vi "Becker-Hickl Read Single SGL.vi"(8 "Error In":errorcluster, 10 "Default":sgl, 11 "Bytes in":string) -> (0 "Error Out":errorcluster, 2 "SGL":sgl, 3 "Bytes out":string)   [LabVIEW 2021, in "Becker-Hickl Files.lvlib"]
uses:
  Becker-Hickl Files.lvlib
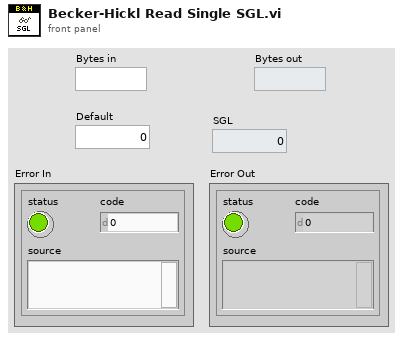
[diagram p1: front panel]
types:
  T1 = enum16{"big-endian, network order", "native, host order", "little-endian"}
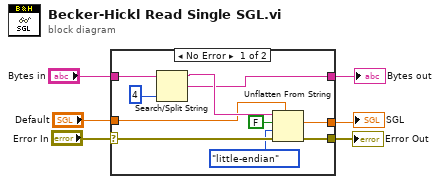
[diagram p0: block diagram]
diagram:
  n1 = case shown="No Error" "Error In" {
    selector: "Error In" -> [w12 w17]
    tunnel: [w13 w18] -> w6
    tunnel: "Bytes in" -> [w16 w18]
    tunnel: [w11 _] -> w3
    tunnel: [w10 w17] -> w2
    tunnel: "Default" -> [w7 _]
    frame No Error {
      n2 = Search/Split String(string=w16, offset (0)=4 ("index")) -> (substring before match=w14:string, match + rest of string=w13:string)  [unwired: 1 in, 1 out]
      n3 = Unflatten From String(type=w7, binary string=w14, data includes array or string size? (T)=FALSE, byte order (0:big-endian, network order)=T1."little-endian", error in (no error)=w12) -> (value=w11:sgl, error out=w10:errorcluster)  [unwired: 1 out]
    }
    frame Error {
    }
  }
  "SGL" <- w3
  "Bytes out" <- w6
  "Error Out" <- w2
